vi "overlay3channels.vi"(6 "active channels":bool[](array[boolean]), 8 "RGB Overlay":T1, 11 "Array":T2(array[cluster])) -> (0 "RGB Image Out":T1)   [LabVIEW 2017]
doc: "SciScan 1.2 160622"
uses:
  <vilib>/vision/Image Controls.llb/IMAQ Image.ctl
  Custom Controls/Ch selector.ctl
  <vilib>/vision/NI_Vision_Development_Module.lvlib
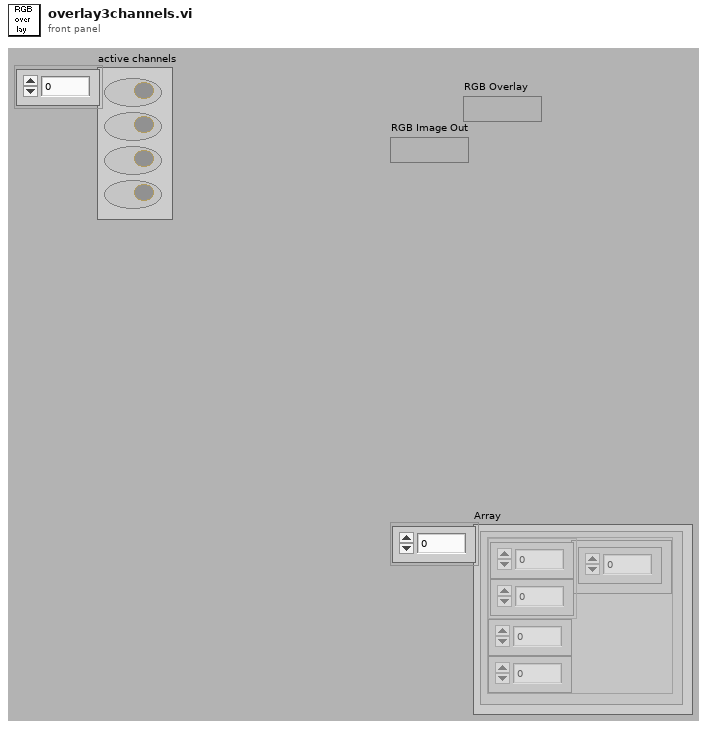
[diagram p1: front panel]
types:
  T1 = typedef "IMAQ Image.ctl" = refnum<image>
  T2 = cluster{"Array":i16[][], "Numeric Control":i32, "Numeric Control":i32}[]
  T3 = typedef "Ch selector.ctl" = enum16{"none", "Ch 1", "Ch 2", "Ch 3", "Ch 4"}
  T4 = cluster{"Array":i16[][], "Numeric Control":i32, "Numeric Control":i32}
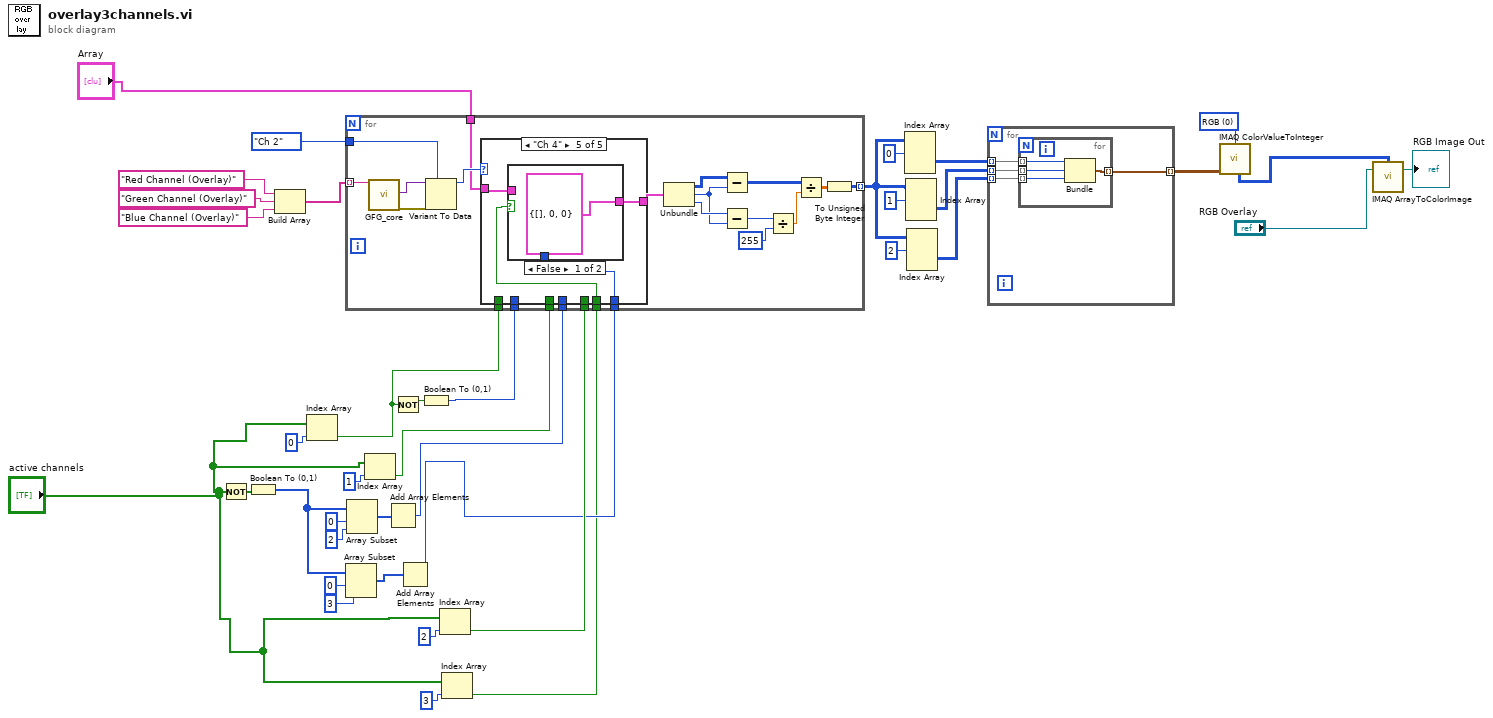
[diagram p0: block diagram]
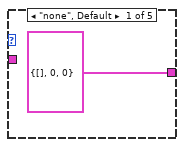
[diagram p2: hidden frame]
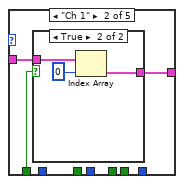
[diagram p3: hidden frame]
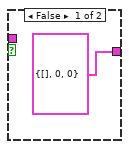
[diagram p4: hidden frame]
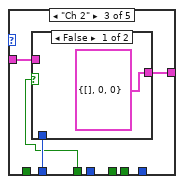
[diagram p5: hidden frame]
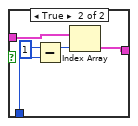
[diagram p6: hidden frame]
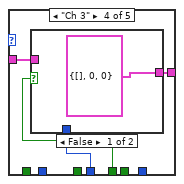
[diagram p7: hidden frame]
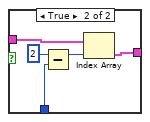
[diagram p8: hidden frame]
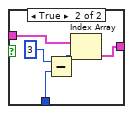
[diagram p9: hidden frame]
diagram:
  w38 = u16 0 items=["RGB", "HSL", "HSV", "HSI"] ("Color Mode")
  n1 = Not(x="active channels") -> (.not. x?=w16:bool[])
  n2 = Boolean To (0,1)(Boolean=w16) -> (0, 1=w17:i16[])
  n3 = Build Array("Red Channel (Overlay)" ("Variable Name in"), "Green Channel (Overlay)" ("Variable Name in"), "Blue Channel (Overlay)" ("Variable Name in")) -> (w32:string[])
  n4 = Index Array(array="active channels", index=0) -> (element=w10:bool)
  n5 = Array Subset(array=w17, index=0, length=3) -> (w14:i16[])
  n6 = Array Subset(array=w17, index=0, length=2) -> (w15:i16[])
  n7 = Index Array(array="active channels", index=1) -> (element=w6:bool)
  n8 = Add Array Elements(numeric array=w15) -> (sum=w4:i16)
  n9 = Not(x=w10) -> (.not. x?=w13:bool)
  n10 = Add Array Elements(numeric array=w14) -> (sum=w3:i16)
  n11 = Boolean To (0,1)(Boolean=w13) -> (0, 1=w9:i16)
  n12 = Index Array(array="active channels", index=2) -> (element=w5:bool)
  n13 = Index Array(array="active channels", index=3) -> (element=w2:bool)
  n14 = for {
    tunnel: w32 -> [w62] mode=indexing
    tunnel: Ch_selector."Ch 2" ("Red Channel (Overlay)") -> [w60]
    tunnel: "Array" -> [w57]
    tunnel: [w48] -> w27 mode=indexing
    tunnel: w10 -> [w46]
    tunnel: w9 -> [w45]
    tunnel: w6 -> [w44]
    tunnel: w5 -> [w43]
    tunnel: w4 -> [w42]
    tunnel: w3 -> [w41]
    tunnel: w2 -> [w40]
    n15 = call "GFG_core.vi"("Variable Name in"=w62) -> ("Variant Out"=w59:variant, "error out"=w61:errorcluster)  [unwired: 12 in, 5 out]
    n16 = Variant To Data(error in=w61, type=w60, Variant=w59) -> (data=w58:T3)  [unwired: 1 out]
    n17 = case shown="\"Ch 4\"" w58 {
      tunnel: w57 -> [_ w66 w74 w84 w94]
      tunnel: [cluster{i16[][], i32, i32} {[], 0, 0} w65 w73 w83 w93] -> w56
      tunnel: w46 -> [_ w64 _ _ _]
      tunnel: w45 -> [_ _ w72 _ _]
      tunnel: w44 -> [_ _ w71 _ _]
      tunnel: w43 -> [_ _ _ w82 _]
      tunnel: w42 -> [_ _ _ w81 _]
      tunnel: w41 -> [_ _ _ _ w92]
      tunnel: w40 -> [_ _ _ _ w91]
      frame "none", Default {
      }
      frame "Ch 1" {
        n18 = case shown="True" w64 {
          tunnel: w66 -> [_ w70]
          tunnel: [cluster{i16[][], i32, i32} {[], 0, 0} w68] -> w65
          frame False {
          }
          frame True {
            n19 = Index Array(array=w70, index=0) -> (element=w68:T4)
          }
        }
      }
      frame "Ch 2" {
        n20 = case shown="False" w71 {
          tunnel: w74 -> [_ w80]
          tunnel: [cluster{i16[][], i32, i32} {[], 0, 0} w78] -> w73
          tunnel: w72 -> [_ w76]
          frame False {
          }
          frame True {
            n21 = Subtract(x=1 ("index"), y=w76) -> (x-y=w77:i32)
            n22 = Index Array(array=w80, index=w77) -> (element=w78:T4)
          }
        }
      }
      frame "Ch 3" {
        n23 = case shown="False" w82 {
          tunnel: w84 -> [_ w90]
          tunnel: [cluster{i16[][], i32, i32} {[], 0, 0} w88] -> w83
          tunnel: w81 -> [_ w86]
          frame False {
          }
          frame True {
            n24 = Subtract(x=2 ("index"), y=w86) -> (x-y=w87:i32)
            n25 = Index Array(array=w90, index=w87) -> (element=w88:T4)
          }
        }
      }
      frame "Ch 4" {
        n26 = case shown="False" w91 {
          tunnel: w94 -> [_ w100]
          tunnel: [cluster{i16[][], i32, i32} {[], 0, 0} w99] -> w93
          tunnel: w92 -> [_ w96]
          frame False {
          }
          frame True {
            n27 = Subtract(x=3 ("index"), y=w96) -> (x-y=w98:i32)
            n28 = Index Array(array=w100, index=w98) -> (element=w99:T4)
          }
        }
      }
    }
    n29 = Unbundle(w56) -> ("Array"=w51:i16[][], "Numeric Control"=w47:i32, "Numeric Control"=w50:i32)
    n30 = Subtract(x=w51, y=w47) -> (x-y=w54:i32[][])
    n31 = Subtract(x=w50, y=w47) -> (x-y=w55:i32)
    n32 = Divide(x=w55, y=i16 255) -> (x/y=w53:dbl)
    n33 = Divide(x=w54, y=w53) -> (x/y=w49:dbl[][])
    n34 = To Unsigned Byte Integer(number=w49) -> (unsigned 8bit integer=w48:u8[][])
  }
  n35 = Index Array(array=w27, index (dim 0)=0 ("index (page)")) -> (element=w25:u8[][])  [unwired: 2 in]
  n36 = Index Array(array=w27, index (dim 0)=1 ("index (page)")) -> (element=w24:u8[][])  [unwired: 2 in]
  n37 = Index Array(array=w27, index (dim 0)=2 ("index (page)")) -> (element=w23:u8[][])  [unwired: 2 in]
  n38 = for {
    tunnel: w25 -> [w102] mode=indexing
    tunnel: [w104] -> w39 mode=indexing
    tunnel: w23 -> [w103] mode=indexing
    tunnel: w24 -> [w101] mode=indexing
    n39 = for {
      tunnel: w102 -> [w108] mode=indexing
      tunnel: [w107] -> w104 mode=indexing
      tunnel: w103 -> [w106] mode=indexing
      tunnel: w101 -> [w105] mode=indexing
      n40 = Bundle(w108, w105, w106) -> (w107:cluster{u8, u8, u8})  [unwired: 1 in]
    }
  }
  n41 = call "IMAQ ColorValueToInteger"("2D Color value array"=w39, "Color Mode"=w38) -> ("2D U32 array"=w37:u32[][])  [unwired: 3 in, 3 out]
  n42 = call "IMAQ ArrayToColorImage"("Image Pixels (U32)"=w37, "Image"="RGB Overlay") -> ("Image Out"=→"RGB Image Out":T1)  [unwired: 3 in, 1 out]
